vi "from_variant_MOVE_MOTION_cmd_data.vi"(11 "variant":variant) -> (2 "target pos":dbl, 3 "OneMotion.lvclass":refnum<class "OneMotion.lvclass">)   [LabVIEW 2016, in "MotionControl_UFO_3DOF.lvlib"]
uses:
  <userlib>/MotionControl_UFO_3DOF/MotionControl_UFO_3DOF.lvlib
  <userlib>/MotionControl_UFO_3DOF/OneMotion/OneMotion.lvclass
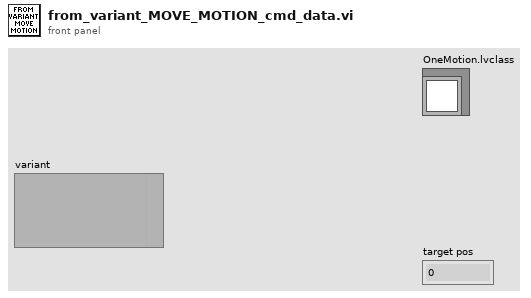
[diagram p1: front panel]
types:
  T1 = cluster{"OneMotion.lvclass 2":refnum<class "OneMotion.lvclass">, dbl}
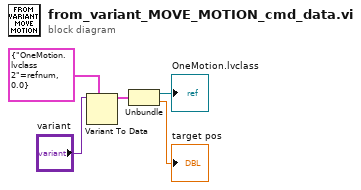
[diagram p0: block diagram]
diagram:
  n1 = Variant To Data(type=T1 {"OneMotion.lvclass 2"=refnum, 0.0}, Variant="variant") -> (data=w3:T1)  [unwired: 1 in, 1 out]
  n2 = Unbundle(w3) -> ("OneMotion.lvclass 2"=→"OneMotion.lvclass":refnum<class "OneMotion.lvclass">, →"target pos":dbl)
